vi "Read (Min Current).vi"(0 "VISA resource name":refnum<visa-resource-name>, 11 "error in (no error)":errorcluster) -> (4 "VISA resource name out":refnum<visa-resource-name>, 6 "Min Current (A)":dbl, 15 "error out":errorcluster)   [LabVIEW 2020, in "NH Research Regenerative Test Series.lvlib"]
doc: "Returns the minimum current in Amperes during the aperture."
uses:
  <instrlib>/NH Research Regenerative Test Series/NH Research Regenerative Test Series.lvlib
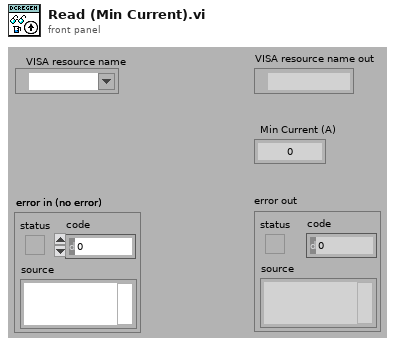
[diagram p1: front panel]
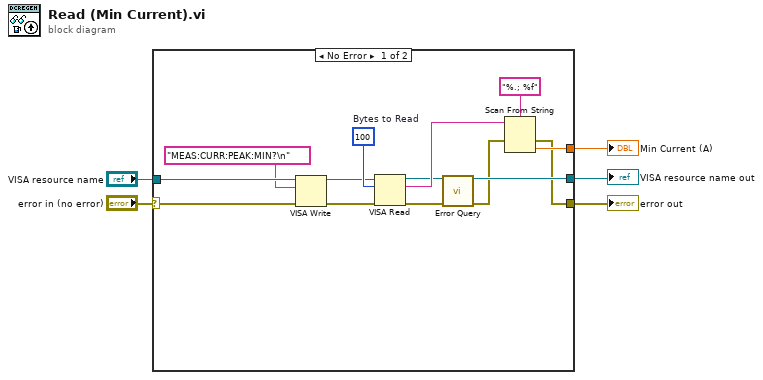
[diagram p0: block diagram]
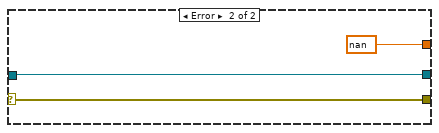
[diagram p2: hidden frame]
diagram:
  n1 = case shown="No Error" "error in (no error)" {
    selector: "error in (no error)" -> [w6 w22]
    tunnel: [w8 w22] -> w4
    tunnel: [w12 w21] -> w2
    tunnel: "VISA resource name" -> [w16 w21]
    tunnel: [w13 nan] -> w1
    frame No Error {
      w19 = u32 100  # Bytes to Read
      n2 = VISA Write(VISA resource name=w16, write buffer="MEAS:CURR:PEAK:MIN?\n" ("Command"), error in (no error)=w6) -> (VISA resource name out=w17:refnum<visa-resource-name>, error out=w18:errorcluster)  [unwired: 1 out]
      n3 = VISA Read(VISA resource name=w17, byte count=w19, error in (no error)=w18) -> (VISA resource name out=w11:refnum<visa-resource-name>, read buffer=w15:string, error out=w10:errorcluster)  [unwired: 1 out]
      n4 = call <instrlib>:"Error Query.vi"("VISA resource name"=w11, "error in (no error)"=w10) -> ("VISA resource name out"=w12:refnum<visa-resource-name>, "error out"=w9:errorcluster)  [unwired: 10 in, 2 out]
      n5 = Scan From String(format string="%.; %f", input string=w15, error in=w9) -> (error out=w8:errorcluster, output 1=w13:dbl)  [unwired: 2 in, 2 out]
    }
    frame Error {
    }
  }
  "error out" <- w4
  "VISA resource name out" <- w2
  "Min Current (A)" <- w1
